vi "Lab Panel V4.91.vi"() -> ()   [LabVIEW 2013] (continued)
                            n2887 = case shown="True" w5366 {
                              tunnel: [w5368 0] -> w5364
                              tunnel: w5363 -> [w5368 _]
                              tunnel: w5365 -> [_ w5369]
                              frame False {
                              }
                              frame True {
                                n2888 = Concatenate Strings("LA02-1 ", w5369) -> (w5372:string)
                                n2889 = One Button Dialog(message=w5372) -> ()  [unwired: 1 in, 1 out]
                              }
                            }
                          }
                          frame #3 {
                            n2890 = Greater?(x=w5374, y=w5377) -> (0:w5376:bool)
                            n2891 = case shown="True" w5376 {
                              tunnel: [w5378 0] -> w5373
                              tunnel: w5374 -> [w5378 _]
                              tunnel: w5375 -> [_ w5379]
                              frame False {
                              }
                              frame True {
                                n2892 = Concatenate Strings("LA02-2 ", w5379) -> (w5382:string)
                                n2893 = One Button Dialog(message=w5382) -> ()  [unwired: 1 in, 1 out]
                              }
                            }
                          }
                          frame #4 {
                            n2894 = Greater?(x=w5384, y=w5387) -> (0:w5386:bool)
                            n2895 = case shown="True" w5386 {
                              tunnel: [w5388 0] -> w5383
                              tunnel: w5384 -> [w5388 _]
                              tunnel: w5385 -> [_ w5389]
                              frame False {
                              }
                              frame True {
                                n2896 = Concatenate Strings("LA03-1 ", w5389) -> (w5392:string)
                                n2897 = One Button Dialog(message=w5392) -> ()  [unwired: 1 in, 1 out]
                              }
                            }
                          }
                          frame #5 {
                            n2898 = Greater?(x=w5393, y=w5397) -> (0:w5396:bool)
                            n2899 = case shown="True" w5396 {
                              tunnel: [w5398 0] -> w5394
                              tunnel: w5393 -> [w5398 _]
                              tunnel: w5395 -> [_ w5399]
                              frame False {
                              }
                              frame True {
                                n2900 = Concatenate Strings("LA03-2 ", w5399) -> (w5402:string)
                                n2901 = One Button Dialog(message=w5402) -> ()  [unwired: 1 in, 1 out]
                              }
                            }
                          }
                          frame #6 {
                            n2902 = Greater?(x=w5404, y=w5407) -> (0:w5406:bool)
                            n2903 = case shown="True" w5406 {
                              tunnel: [w5408 0] -> w5403
                              tunnel: w5404 -> [w5408 _]
                              tunnel: w5405 -> [_ w5409]
                              frame False {
                              }
                              frame True {
                                n2904 = Concatenate Strings("LA04-1 ", w5409) -> (w5412:string)
                                n2905 = One Button Dialog(message=w5412) -> ()  [unwired: 1 in, 1 out]
                              }
                            }
                          }
                          frame #7 {
                            n2906 = Greater?(x=w5414, y=w5417) -> (0:w5416:bool)
                            n2907 = case shown="True" w5416 {
                              tunnel: [w5418 0] -> w5413
                              tunnel: w5414 -> [w5418 _]
                              tunnel: w5415 -> [_ w5419]
                              frame False {
                              }
                              frame True {
                                n2908 = Concatenate Strings("LA04-2 ", w5419) -> (w5422:string)
                                n2909 = One Button Dialog(message=w5422) -> ()  [unwired: 1 in, 1 out]
                              }
                            }
                          }
                          frame #8 {
                            n2910 = Greater?(x=w5424, y=w5427) -> (0:w5426:bool)
                            n2911 = case shown="True" w5426 {
                              tunnel: [w5428 0] -> w5423
                              tunnel: w5424 -> [w5428 _]
                              tunnel: w5425 -> [_ w5429]
                              frame False {
                              }
                              frame True {
                                n2912 = Concatenate Strings("LA05-1 ", w5429) -> (w5432:string)
                                n2913 = One Button Dialog(message=w5432) -> ()  [unwired: 1 in, 1 out]
                              }
                            }
                          }
                          frame #9 {
                            n2914 = Greater?(x=w5434, y=w5437) -> (0:w5436:bool)
                            n2915 = case shown="True" w5436 {
                              tunnel: [w5438 0] -> w5433
                              tunnel: w5434 -> [w5438 _]
                              tunnel: w5435 -> [_ w5439]
                              frame False {
                              }
                              frame True {
                                n2916 = Concatenate Strings("LA05-2 ", w5439) -> (w5442:string)
                                n2917 = One Button Dialog(message=w5442) -> ()  [unwired: 1 in, 1 out]
                              }
                            }
                          }
                        }
                        n2918 = Bundle By Name(cluster=w5341, "LAB01-1"=w5339, "LAB01-2"=w5337, "LAB02-1"=w5334, "LAB02-2"=w5331, "LAB03-1"=w5329, "LAB03-2"=w5328, "LAB04-1"=w5325, "LAB04-2"=w5323, "LAB05-1"=w5321, "LAB05-2"=w5319) -> (w5340:T8)
                        n2919 = local write "JIG RELAY CYCLES"(w5340) -> ()
                      }
                    }
                  }
                }
              }
            }
          }
          frame #19 {
            # "get temperature values"
            n2920 = local read "Panel #"() -> (w5443:dbl)
            n2921 = local read "simulate"() -> (w5456:bool)
            n2922 = local read "Temp Test Cal"() -> (w5453:dbl)
            n2923 = stacked-sequence {
              seq-local: [w5459 _] -> [_ w5495]
              tunnel: w5456 -> [_ w5509]
              tunnel: T14 {"1  (A) cal"=1.0, "1 (V) cal"=1.0, "1 (PF) cal"=1.0, "1 (TL) cal"=1.0, "1 (TN) cal"=1.0, "2 (A) cal"=1.0, "2 (V) cal"=1.0, "2 (PF) cal"=1.0, "2 (TL) cal"=1.0, "2 (TN) cal"=1.0} ("CAL LAB01") -> [_ w5508]
              tunnel: w5454 -> [_ w5507]
              tunnel: w5453 -> [_ w5506]
              tunnel: w5452 -> [_ w5505]
              tunnel: w5451 -> [_ w5504]
              tunnel: w5450 -> [_ w5503]
              tunnel: w5449 -> [_ w5502]
              tunnel: w5448 -> [_ w5501]
              tunnel: w5447 -> [_ w5500]
              tunnel: w5446 -> [_ w5499]
              tunnel: w5445 -> [_ w5498]
              tunnel: w5444 -> [_ w5497]
              tunnel: w5443 -> [_ w5496]
              frame #0 {
                n2924 = local read "Select COM port"() -> (w5460:refnum<visa-resource-name>)
                "COM port" <- w5460
                n2925 = global write "Global 1.vi" "COM port"(w5460) -> ()
                n2926 = global write "Global 1.vi" "tmp dly lps"("Temp Delay Lps") -> ()
                n2927 = global write "Global 1.vi" "dly value"("Temp Value") -> ()
                n2928 = local read "jig cycle"() -> (w5462:dbl)
                n2929 = local read "on loops"() -> (w5464:dbl)
                n2930 = Add(x=w5464, y=3) -> (x+y=w5465:dbl)
                n2931 = local read "Panel #"() -> (w5461:dbl)
                n2932 = Equal?(x=w5462, y=w5465) -> (x = y?=w5459:bool)
                n2933 = case shown="True" w5459 {
                  tunnel: w5461 -> [_ w5469]
                  frame False {
                  }
                  frame True {
                    n2934 = local read "simulate"() -> (w5466:bool)
                    n2935 = case shown="1" w5469 {
                      tunnel: 1.0 -> [_ w5474 w5476 w5482 w5486 w5491]
                      tunnel: w5466 -> [_ w5470 w5475 w5480 w5487 w5490]
                      frame 0, Default {
                      }
                      frame 1 {
                        w5472 = FALSE
                        n2936 = call "sub vi - GET ALL TEMP v6.vi"("LA01-EN"=TRUE, "simulate"=w5470, "LA02-EN"=w5472, "LA03-EN"=w5472, "LA04-EN"=w5472, "LA05-EN"=w5472, "Gen Cal Value"=w5474) -> ("LA01 TEMP"=w5471:T24)  [unwired: 3 in, 5 out]
                        n2937 = local write "LAB01 TEMP"(w5471) -> ()
                      }
                      frame 2 {
                        w5477 = FALSE
                        n2938 = call "sub vi - GET ALL TEMP v6.vi"("LA01-EN"=w5477, "simulate"=w5475, "LA02-EN"=TRUE, "LA03-EN"=w5477, "LA04-EN"=w5477, "LA05-EN"=w5477, "Gen Cal Value"=w5476) -> ("LA02 TEMP"=w5479:T24)  [unwired: 3 in, 5 out]
                        n2939 = local write "LAB02 TEMP"(w5479) -> ()
                      }
                      frame 3 {
                        w5483 = FALSE
                        n2940 = call "sub vi - GET ALL TEMP v6.vi"("LA01-EN"=w5483, "simulate"=w5480, "LA02-EN"=w5483, "LA03-EN"=TRUE, "LA04-EN"=w5483, "LA05-EN"=w5483, "Gen Cal Value"=w5482) -> ("LA03 TEMP"=w5481:T24)  [unwired: 3 in, 5 out]
                        n2941 = local write "LAB03 TEMP"(w5481) -> ()
                      }
                      frame 4 {
                        w5488 = FALSE
                        n2942 = call "sub vi - GET ALL TEMP v6.vi"("LA01-EN"=w5488, "simulate"=w5487, "LA02-EN"=w5488, "LA03-EN"=w5488, "LA04-EN"=TRUE, "LA05-EN"=w5488, "Gen Cal Value"=w5486) -> ("LA04 TEMP"=w5485:T24)  [unwired: 3 in, 5 out]
                        n2943 = local write "LAB04 TEMP"(w5485) -> ()
                      }
                      frame 5 {
                        w5493 = FALSE
                        n2944 = call "sub vi - GET ALL TEMP v6.vi"("LA01-EN"=w5493, "simulate"=w5490, "LA02-EN"=w5493, "LA03-EN"=w5493, "LA04-EN"=w5493, "LA05-EN"=TRUE, "Gen Cal Value"=w5491) -> ("LA05 TEMP"=w5492:T24)  [unwired: 3 in, 5 out]
                        n2945 = local write "LAB05 TEMP"(w5492) -> ()
                      }
                    }
                    n2946 = local write "TEMP"(TRUE) -> ()
                  }
                }
              }
              frame #1 {
                n2947 = case shown="True" w5495 {
                  tunnel: w5509 -> [_ w5523]
                  tunnel: w5508 -> [_ w5522]
                  tunnel: w5507 -> [_ w5521]
                  tunnel: w5506 -> [_ w5520]
                  tunnel: w5505 -> [_ w5519]
                  tunnel: w5504 -> [_ w5518]
                  tunnel: w5503 -> [_ w5517]
                  tunnel: w5502 -> [_ w5516]
                  tunnel: w5501 -> [_ w5515]
                  tunnel: w5500 -> [_ w5514]
                  tunnel: w5499 -> [_ w5513]
                  tunnel: w5498 -> [_ w5512]
                  tunnel: w5497 -> [_ w5511]
                  tunnel: w5496 -> [_ w5510]
                  frame False {
                  }
                  frame True {
                    n2948 = case shown="1" w5510 {
                      tunnel: w5523 -> [_ w5536 w5581 w5626 w5671 w5716]
                      tunnel: w5522 -> [_ w5535 w5580 w5625 w5670 w5715]
                      tunnel: w5521 -> [_ w5525 _ _ _ _]
                      tunnel: w5520 -> [_ w5530 w5579 w5624 w5669 w5714]
                      tunnel: w5519 -> [_ w5524 _ _ _ _]
                      tunnel: w5518 -> [_ _ w5570 _ _ _]
                      tunnel: w5517 -> [_ _ w5569 _ _ _]
                      tunnel: w5516 -> [_ _ _ w5615 _ _]
                      tunnel: w5515 -> [_ _ _ w5614 _ _]
                      tunnel: w5514 -> [_ _ _ _ w5660 _]
                      tunnel: w5513 -> [_ _ _ _ w5659 _]
                      tunnel: w5512 -> [_ _ _ _ _ w5705]
                      tunnel: w5511 -> [_ _ _ _ _ w5704]
                      frame ..0 {
                      }
                      frame 1 {
                        n2949 = case shown="False" w5536 {
                          tunnel: [w5567 w5568] -> w5552
                          tunnel: w5535 -> [_ w5568]
                          frame False {
                            n2950 = local read "CAL LAB01"() -> (w5567:T14)
                          }
                          frame True {
                          }
                        }
                        n2951 = local read "TEMP LA01"() -> (w5543:T9)
                        n2952 = local read "LAB01 TEMP"() -> (w5542:T12)
                        n2953 = call "sub vi - temperature delay v3.vi"("2-run"=w5524, "1-run"=w5525, "temp values IN"=w5543, "temp signals"=w5542) -> ("T2-N"=w5538:dbl, "T2-L"=w5539:dbl, "T1-N"=w5540:dbl, "T1-L"=w5541:dbl, "temp values OUT"=w5537:T43)  [unwired: 3 in]
                        n2954 = Unbundle By Name(w5552) -> ("1 (TL) cal"=w5547:dbl, "1 (TN) cal"=w5546:dbl, "2 (TL) cal"=w5545:dbl, "2 (TN) cal"=w5544:dbl)  [unwired: 6 out]
                        n2955 = local write "TEMP LA01"(w5537) -> ()
                        n2956 = Multiply(x=w5541, y=w5547) -> (x*y=w5534:dbl)
                        n2957 = Multiply(x=w5540, y=w5546) -> (x*y=w5532:dbl)
                        n2958 = Multiply(x=w5539, y=w5545) -> (x*y=w5529:dbl)
                        n2959 = Multiply(x=w5538, y=w5544) -> (x*y=w5528:dbl)
                        n2960 = case shown="True" w5525 {
                          tunnel: w5534 -> [w5561 w5566]
                          tunnel: w5530 -> [_ w5564]
                          tunnel: [w5561 w5565] -> w5533
                          tunnel: w5532 -> [w5560 w5563]
                          tunnel: [w5560 w5562] -> w5531
                          frame False {
                          }
                          frame True {
                            n2961 = Multiply(x=w5564, y=w5563) -> (x*y=w5562:dbl)
                            n2962 = Multiply(x=w5564, y=w5566) -> (x*y=w5565:dbl)
                          }
                        }
                        n2963 = case shown="True" w5524 {
                          tunnel: w5529 -> [w5554 w5559]
                          tunnel: w5530 -> [_ w5557]
                          tunnel: [w5554 w5558] -> w5527
                          tunnel: w5528 -> [w5553 w5556]
                          tunnel: [w5553 w5555] -> w5526
                          frame False {
                          }
                          frame True {
                            n2964 = Multiply(x=w5557, y=w5556) -> (x*y=w5555:dbl)
                            n2965 = Multiply(x=w5557, y=w5559) -> (x*y=w5558:dbl)
                          }
                        }
                        n2966 = local read "SIG LAB01-2"() -> (w5549:T2)
                        n2967 = local read "SIG LAB01-1"() -> (w5551:T2)
                        n2968 = Bundle By Name(cluster=w5551, "Tmp Live"=w5533, "Tmp Neut"=w5531) -> (w5550:T2)
                        n2969 = Bundle By Name(cluster=w5549, "Tmp Live"=w5527, "Tmp Neut"=w5526) -> (w5548:T2)
                        n2970 = local write "SIG LAB01-1"(w5550) -> ()
                        n2971 = local write "SIG LAB01-2"(w5548) -> ()
                      }
                      frame 2 {
                        n2972 = case shown="True" w5581 {
                          tunnel: [w5612 w5613] -> w5597
                          tunnel: w5580 -> [_ w5613]
                          frame False {
                            n2973 = local read "CAL LAB02"() -> (w5612:T15)
                          }
                          frame True {
                          }
                        }
                        n2974 = local read "LAB02 TEMP"() -> (w5588:T12)
                        n2975 = local read "TEMP LA02"() -> (w5587:T9)
                        n2976 = call "sub vi - temperature delay v3.vi"("2-run"=w5569, "1-run"=w5570, "temp values IN"=w5587, "temp signals"=w5588) -> ("T2-N"=w5582:dbl, "T2-L"=w5583:dbl, "T1-N"=w5584:dbl, "T1-L"=w5585:dbl, "temp values OUT"=w5586:T43)  [unwired: 3 in]
                        n2977 = Unbundle By Name(w5597) -> ("1 (TL) cal"=w5592:dbl, "1 (TN) cal"=w5591:dbl, "2 (TL) cal"=w5590:dbl, "2 (TN) cal"=w5589:dbl)  [unwired: 6 out]
                        n2978 = local write "TEMP LA02"(w5586) -> ()
                        n2979 = Multiply(x=w5585, y=w5592) -> (x*y=w5578:dbl)
                        n2980 = Multiply(x=w5584, y=w5591) -> (x*y=w5577:dbl)
                        n2981 = Multiply(x=w5583, y=w5590) -> (x*y=w5574:dbl)
                        n2982 = Multiply(x=w5582, y=w5589) -> (x*y=w5573:dbl)
                        n2983 = case shown="True" w5570 {
                          tunnel: w5578 -> [w5606 w5611]
                          tunnel: w5579 -> [_ w5609]
                          tunnel: [w5606 w5610] -> w5576
                          tunnel: w5577 -> [w5605 w5608]
                          tunnel: [w5605 w5607] -> w5575
                          frame False {
                          }
                          frame True {
                            n2984 = Multiply(x=w5609, y=w5608) -> (x*y=w5607:dbl)
                            n2985 = Multiply(x=w5609, y=w5611) -> (x*y=w5610:dbl)
                          }
                        }
                        n2986 = case shown="True" w5569 {
                          tunnel: w5574 -> [w5599 w5604]
                          tunnel: w5579 -> [_ w5602]
                          tunnel: [w5599 w5603] -> w5572
                          tunnel: w5573 -> [w5598 w5601]
                          tunnel: [w5598 w5600] -> w5571
                          frame False {
                          }
                          frame True {
                            n2987 = Multiply(x=w5602, y=w5601) -> (x*y=w5600:dbl)
                            n2988 = Multiply(x=w5602, y=w5604) -> (x*y=w5603:dbl)
                          }
                        }
                        n2989 = local read "SIG LAB02-2"() -> (w5594:T2)
                        n2990 = local read "SIG LAB02-1"() -> (w5596:T2)
                        n2991 = Bundle By Name(cluster=w5596, "Tmp Live"=w5576, "Tmp Neut"=w5575) -> (w5595:T2)
                        n2992 = Bundle By Name(cluster=w5594, "Tmp Live"=w5572, "Tmp Neut"=w5571) -> (w5593:T2)
                        n2993 = local write "SIG LAB02-1"(w5595) -> ()
                        n2994 = local write "SIG LAB02-2"(w5593) -> ()
                      }
                      frame 3 {
                        n2995 = case shown="False" w5626 {
                          tunnel: [w5657 w5658] -> w5642
                          tunnel: w5625 -> [_ w5658]
                          frame False {
                            n2996 = local read "CAL LAB03"() -> (w5657:T14)
                          }
                          frame True {
                          }
                        }
                        n2997 = local read "TEMP LA03"() -> (w5632:T9)
                        n2998 = local read "LAB03 TEMP"() -> (w5633:T12)
                        n2999 = call "sub vi - temperature delay v3.vi"("2-run"=w5614, "1-run"=w5615, "temp values IN"=w5632, "temp signals"=w5633) -> ("T2-N"=w5627:dbl, "T2-L"=w5628:dbl, "T1-N"=w5629:dbl, "T1-L"=w5630:dbl, "temp values OUT"=w5631:T43)  [unwired: 3 in]
                        n3000 = Unbundle By Name(w5642) -> ("1 (TL) cal"=w5637:dbl, "1 (TN) cal"=w5636:dbl, "2 (TL) cal"=w5635:dbl, "2 (TN) cal"=w5634:dbl)  [unwired: 6 out]
                        n3001 = local write "TEMP LA03"(w5631) -> ()
                        n3002 = Multiply(x=w5630, y=w5637) -> (x*y=w5623:dbl)
                        n3003 = Multiply(x=w5629, y=w5636) -> (x*y=w5622:dbl)
                        n3004 = Multiply(x=w5628, y=w5635) -> (x*y=w5619:dbl)
                        n3005 = Multiply(x=w5627, y=w5634) -> (x*y=w5618:dbl)
                        n3006 = case shown="True" w5614 {
                          tunnel: w5619 -> [w5644 w5649]
                          tunnel: w5624 -> [_ w5647]
                          tunnel: [w5644 w5648] -> w5617
                          tunnel: w5618 -> [w5643 w5646]
                          tunnel: [w5643 w5645] -> w5616
                          frame False {
                          }
                          frame True {
                            n3007 = Multiply(x=w5647, y=w5646) -> (x*y=w5645:dbl)
                            n3008 = Multiply(x=w5647, y=w5649) -> (x*y=w5648:dbl)
                          }
                        }
                        n3009 = case shown="True" w5615 {
                          tunnel: w5623 -> [w5651 w5656]
                          tunnel: w5624 -> [_ w5654]
                          tunnel: [w5651 w5655] -> w5621
                          tunnel: w5622 -> [w5650 w5653]
                          tunnel: [w5650 w5652] -> w5620
                          frame False {
                          }
                          frame True {
                            n3010 = Multiply(x=w5654, y=w5653) -> (x*y=w5652:dbl)
                            n3011 = Multiply(x=w5654, y=w5656) -> (x*y=w5655:dbl)
                          }
                        }
                        n3012 = local read "SIG LAB03-2"() -> (w5639:T2)
                        n3013 = local read "SIG LAB03-1"() -> (w5641:T2)
                        n3014 = Bundle By Name(cluster=w5641, "Tmp Live"=w5621, "Tmp Neut"=w5620) -> (w5640:T2)
                        n3015 = Bundle By Name(cluster=w5639, "Tmp Live"=w5617, "Tmp Neut"=w5616) -> (w5638:T2)
                        n3016 = local write "SIG LAB03-1"(w5640) -> ()
                        n3017 = local write "SIG LAB03-2"(w5638) -> ()
                      }
                      frame 4 {
                        n3018 = case shown="False" w5671 {
                          tunnel: [w5702 w5703] -> w5687
                          tunnel: w5670 -> [_ w5703]
                          frame False {
                            n3019 = local read "CAL LAB04"() -> (w5702:T14)
                          }
                          frame True {
                          }
                        }
                        n3020 = local read "LAB04 TEMP"() -> (w5677:T12)
                        n3021 = local read "TEMP LA04"() -> (w5678:T9)
                        n3022 = call "sub vi - temperature delay v3.vi"("2-run"=w5659, "1-run"=w5660, "temp values IN"=w5678, "temp signals"=w5677) -> ("T2-N"=w5672:dbl, "T2-L"=w5673:dbl, "T1-N"=w5674:dbl, "T1-L"=w5675:dbl, "temp values OUT"=w5676:T43)  [unwired: 3 in]
                        n3023 = Unbundle By Name(w5687) -> ("1 (TL) cal"=w5682:dbl, "1 (TN) cal"=w5681:dbl, "2 (TL) cal"=w5680:dbl, "2 (TN) cal"=w5679:dbl)  [unwired: 6 out]
                        n3024 = local write "TEMP LA04"(w5676) -> ()
                        n3025 = Multiply(x=w5675, y=w5682) -> (x*y=w5668:dbl)
                        n3026 = Multiply(x=w5674, y=w5681) -> (x*y=w5667:dbl)
                        n3027 = Multiply(x=w5673, y=w5680) -> (x*y=w5664:dbl)
                        n3028 = Multiply(x=w5672, y=w5679) -> (x*y=w5663:dbl)
                        n3029 = case shown="True" w5659 {
                          tunnel: w5664 -> [w5689 w5694]
                          tunnel: w5669 -> [_ w5692]
                          tunnel: [w5689 w5693] -> w5662
                          tunnel: w5663 -> [w5688 w5691]
                          tunnel: [w5688 w5690] -> w5661
                          frame False {
                          }
                          frame True {
                            n3030 = Multiply(x=w5692, y=w5691) -> (x*y=w5690:dbl)
                            n3031 = Multiply(x=w5692, y=w5694) -> (x*y=w5693:dbl)
                          }
                        }
                        n3032 = case shown="True" w5660 {
                          tunnel: w5668 -> [w5696 w5701]
                          tunnel: w5669 -> [_ w5699]
                          tunnel: [w5696 w5700] -> w5666
                          tunnel: w5667 -> [w5695 w5698]
                          tunnel: [w5695 w5697] -> w5665
                          frame False {
                          }
                          frame True {
                            n3033 = Multiply(x=w5699, y=w5698) -> (x*y=w5697:dbl)
                            n3034 = Multiply(x=w5699, y=w5701) -> (x*y=w5700:dbl)
                          }
                        }
                        n3035 = local read "SIG LAB04-2"() -> (w5684:T2)
                        n3036 = local read "SIG LAB04-1"() -> (w5686:T2)
                        n3037 = Bundle By Name(cluster=w5686, "Tmp Live"=w5666, "Tmp Neut"=w5665) -> (w5685:T2)
                        n3038 = Bundle By Name(cluster=w5684, "Tmp Live"=w5662, "Tmp Neut"=w5661) -> (w5683:T2)
                        n3039 = local write "SIG LAB04-1"(w5685) -> ()
                        n3040 = local write "SIG LAB04-2"(w5683) -> ()
                      }
                      frame 5.. {
                        n3041 = case shown="False" w5716 {
                          tunnel: [w5747 w5748] -> w5732
                          tunnel: w5715 -> [_ w5748]
                          frame False {
                            n3042 = local read "CAL LAB05"() -> (w5747:T14)
                          }
                          frame True {
                          }
                        }
                        n3043 = local read "LAB05 TEMP"() -> (w5722:T12)
                        n3044 = local read "TEMP LA05"() -> (w5723:T9)
                        n3045 = call "sub vi - temperature delay v3.vi"("2-run"=w5704, "1-run"=w5705, "temp values IN"=w5723, "temp signals"=w5722) -> ("T2-N"=w5718:dbl, "T2-L"=w5719:dbl, "T1-N"=w5720:dbl, "T1-L"=w5721:dbl, "temp values OUT"=w5717:T43)  [unwired: 3 in]
                        n3046 = local write "TEMP LA05"(w5717) -> ()
                        n3047 = Unbundle By Name(w5732) -> ("1 (TL) cal"=w5724:dbl, "1 (TN) cal"=w5727:dbl, "2 (TL) cal"=w5726:dbl, "2 (TN) cal"=w5725:dbl)  [unwired: 6 out]
                        n3048 = Multiply(x=w5721, y=w5724) -> (x*y=w5713:dbl)
                        n3049 = Multiply(x=w5720, y=w5727) -> (x*y=w5712:dbl)
                        n3050 = Multiply(x=w5719, y=w5726) -> (x*y=w5709:dbl)
                        n3051 = Multiply(x=w5718, y=w5725) -> (x*y=w5708:dbl)
                        n3052 = case shown="True" w5704 {
                          tunnel: w5709 -> [w5734 w5739]
                          tunnel: w5714 -> [_ w5737]
                          tunnel: [w5734 w5738] -> w5707
                          tunnel: w5708 -> [w5733 w5736]
                          tunnel: [w5733 w5735] -> w5706
                          frame False {
                          }
                          frame True {
                            n3053 = Multiply(x=w5737, y=w5736) -> (x*y=w5735:dbl)
                            n3054 = Multiply(x=w5737, y=w5739) -> (x*y=w5738:dbl)
                          }
                        }
                        n3055 = case shown="True" w5705 {
                          tunnel: w5713 -> [w5741 w5746]
                          tunnel: w5714 -> [_ w5744]
                          tunnel: [w5741 w5745] -> w5711
                          tunnel: w5712 -> [w5740 w5743]
                          tunnel: [w5740 w5742] -> w5710
                          frame False {
                          }
                          frame True {
                            n3056 = Multiply(x=w5744, y=w5743) -> (x*y=w5742:dbl)
                            n3057 = Multiply(x=w5744, y=w5746) -> (x*y=w5745:dbl)
                          }
                        }
                        n3058 = local read "SIG LAB05-1"() -> (w5731:T2)
                        n3059 = Bundle By Name(cluster=w5731, "Tmp Live"=w5711, "Tmp Neut"=w5710) -> (w5730:T2)
                        n3060 = local read "SIG LAB05-2"() -> (w5729:T2)
                        n3061 = Bundle By Name(cluster=w5729, "Tmp Live"=w5707, "Tmp Neut"=w5706) -> (w5728:T2)
                        n3062 = local write "SIG LAB05-1"(w5730) -> ()
                        n3063 = local write "SIG LAB05-2"(w5728) -> ()
                      }
                    }
                  }
                }
              }
            }
          }
          frame #20 {
            # "write data to display panel"
            n3064 = global write "Global display 1.vi" "TEST 5-2"(w5783) -> ()
            n3065 = global write "Global display 1.vi" "TEST 4-2"(w5785) -> ()
            n3066 = global write "Global display 1.vi" "TEST 1-2"(w5791) -> ()
            n3067 = global write "Global display 1.vi" "TEST 3-1"(w5788) -> ()
            n3068 = global write "Global display 1.vi" "TEST 5-1"(w5784) -> ()
            n3069 = global write "Global display 1.vi" "TEST 1-1"(w5792) -> ()
            n3070 = global write "Global display 1.vi" "TEST 3-2"(w5787) -> ()
            n3071 = global write "Global display 1.vi" "TEST 4-1"(w5786) -> ()
            n3072 = global write "Global display 1.vi" "TEST 2-2"(w5789) -> ()
            n3073 = global write "Global display 1.vi" "TEST 2-1"(w5790) -> ()
            n3074 = global read "Global display 3.vi" "log 1-1"() -> (→"LOG LAB01-1":string)
            n3075 = global read "Global display 3.vi" "log 3-1"() -> (→"LOG LAB03-1":string)
            n3076 = global read "Global display 3.vi" "log 1-2"() -> (→"LOG LAB01-2":string)
            n3077 = property on="Tab Control 2" class="TabCtl (strict)"() -> ("Pages"=w5782:refnum<vi>[])  [unwired: 2 in, 2 out]
            n3078 = global read "Global display 3.vi" "log 2-1"() -> (→"LOG LAB02-1":string)
            n3079 = global read "Global display 3.vi" "log 2-2"() -> (→"LOG LAB02-2":string)
            n3080 = global read "Global display 3.vi" "log 4-2"() -> (→"LOG LAB04-2":string)
            n3081 = global read "Global display 3.vi" "log 5-2"() -> (→"LOG LAB05-2":string)
            n3082 = global read "Global display 3.vi" "log 5-1"() -> (→"LOG LAB05-1":string)
            n3083 = global read "Global display 3.vi" "log 4-1"() -> (→"LOG LAB04-1":string)
            n3084 = global read "Global display 3.vi" "log 3-2"() -> (→"LOG LAB03-2":string)
            n3085 = Index Array(array=w5782, index=8) -> (element=w5780:refnum<vi>)
            n3086 = property class="Page"(reference=w5780) -> ("PageVis"=w5779:bool)  [unwired: 1 in, 2 out]
            n3087 = global write "Global display 3.vi" "admin"(w5779) -> ()
            n3088 = local read "O/I  LAB05-2"() -> (w5833:bool)
            n3089 = local read "O/I  LAB05-1"() -> (w5834:bool)
            n3090 = local read "O/I  LAB03-2"() -> (w5837:bool)
            n3091 = local read "O/I  LAB04-2"() -> (w5835:bool)
            n3092 = local read "O/I  LAB04-1"() -> (w5836:bool)
            n3093 = local read "O/I  LAB03-1"() -> (w5838:bool)
            n3094 = local read "O/I  LAB01-2"() -> (w5841:bool)
            n3095 = local read "O/I  LAB01-1"() -> (w5842:bool)
            n3096 = local read "O/I  LAB02-1"() -> (w5840:bool)
            n3097 = local read "O/I  LAB02-2"() -> (w5839:bool)
            n3098 = global write "Global display 1.vi" "5-2 O/F"(w5833) -> ()
            n3099 = global write "Global display 1.vi" "5-1 O/F"(w5834) -> ()
            n3100 = global write "Global display 1.vi" "4-1 O/F"(w5836) -> ()
            n3101 = global write "Global display 1.vi" "4-2 O/F"(w5835) -> ()
            n3102 = global write "Global display 1.vi" "3-2 O/F"(w5837) -> ()
            n3103 = global write "Global display 1.vi" "3-1 O/F"(w5838) -> ()
            n3104 = global write "Global display 1.vi" "2-2 O/F"(w5839) -> ()
            n3105 = global write "Global display 1.vi" "2-1 O/F"(w5840) -> ()
            n3106 = global write "Global display 1.vi" "1-2 O/F"(w5841) -> ()
            n3107 = global write "Global display 1.vi" "1-1 O/F"(w5842) -> ()
            n3108 = local read "TEMP START LAB02-2"() -> (w5765:cluster{"TL":dbl, "TN":dbl})
            n3109 = local read "run lab05-2"() -> (w5823:bool)
            n3110 = local read "TEMP START LAB01-2"() -> (w5767:cluster{"TL":dbl, "TN":dbl})
            n3111 = local read "TEMP START LAB02-1"() -> (w5766:cluster{"TL":dbl, "TN":dbl})
            n3112 = local read "TEMP START LAB04-1"() -> (w5762:cluster{"TL":dbl, "TN":dbl})
            n3113 = local read "TEMP START LAB04-2"() -> (w5761:cluster{"TL":dbl, "TN":dbl})
            n3114 = local read "run lab04-1"() -> (w5826:bool)
            n3115 = local read "run lab04-2"() -> (w5825:bool)
            n3116 = local read "run lab05-1"() -> (w5824:bool)
            n3117 = local read "TEMP START LAB01-1"() -> (w5768:cluster{"TL":dbl, "TN":dbl})
            n3118 = local read "TEMP START LAB05-2"() -> (w5759:cluster{"TL":dbl, "TN":dbl})
            n3119 = local read "TEMP START LAB05-1"() -> (w5760:cluster{"TL":dbl, "TN":dbl})
            n3120 = local read "run lab03-2"() -> (w5827:bool)
            n3121 = local read "TEMP START LAB03-2"() -> (w5763:cluster{"TL":dbl, "TN":dbl})
            n3122 = local read "TEMP START LAB03-1"() -> (w5764:cluster{"TL":dbl, "TN":dbl})
            n3123 = local read "run lab02-1"() -> (w5830:bool)
            n3124 = local read "run lab03-1"() -> (w5828:bool)
            n3125 = local read "run lab01-2"() -> (w5831:bool)
            n3126 = local read "run lab02-2"() -> (w5829:bool)
            n3127 = local read "run lab01-1"() -> (w5832:bool)
            n3128 = global write "Global display 1.vi" "5-2 R/S"(w5823) -> ()
            n3129 = global write "Global display 1.vi" "5-1 R/S"(w5824) -> ()
            n3130 = global write "Global display 1.vi" "4-2 R/S"(w5825) -> ()
            n3131 = global write "Global display 1.vi" "4-1 R/S"(w5826) -> ()
            n3132 = global write "Global display 1.vi" "3-2 R/S"(w5827) -> ()
            n3133 = global write "Global display 1.vi" "1-2 R/S"(w5831) -> ()
            n3134 = global write "Global display 1.vi" "2-1 R/S"(w5830) -> ()
            n3135 = global write "Global display 1.vi" "3-1 R/S"(w5828) -> ()
            n3136 = global write "Global display 1.vi" "2-2 R/S"(w5829) -> ()
            n3137 = global write "Global display 1.vi" "1-1 R/S"(w5832) -> ()
            n3138 = global write "Global display 3.vi" "TEMP ST 05-2"(w5759) -> ()
            n3139 = global write "Global display 3.vi" "TEMP ST 05-1"(w5760) -> ()
            n3140 = global write "Global display 3.vi" "TEMP ST 03-2"(w5763) -> ()
            n3141 = global write "Global display 3.vi" "TEMP ST 04-2"(w5761) -> ()
            n3142 = global write "Global display 3.vi" "TEMP ST 01-1"(w5768) -> ()
            n3143 = global write "Global display 3.vi" "TEMP ST 01-2"(w5767) -> ()
            n3144 = global write "Global display 3.vi" "TEMP ST 04-1"(w5762) -> ()
            n3145 = global write "Global display 3.vi" "TEMP ST 02-1"(w5766) -> ()
            n3146 = global write "Global display 3.vi" "TEMP ST 02-2"(w5765) -> ()
            n3147 = global write "Global display 3.vi" "TEMP ST 03-1"(w5764) -> ()
            n3148 = local read "DISP LAB04-2"() -> (w5815:T4)
            n3149 = local read "DISP LAB05-1"() -> (w5814:T4)
            n3150 = local read "DISP LAB04-1"() -> (w5816:T4)
            n3151 = local read "DISP LAB05-2"() -> (w5813:T4)
            n3152 = local read "DISP LAB03-1"() -> (w5818:T4)
            n3153 = local read "DISP LAB03-2"() -> (w5817:T4)
            n3154 = local read "DISP LAB01-2"() -> (w5821:T4)
            n3155 = local read "DISP LAB02-1"() -> (w5820:T4)
            n3156 = local read "DISP LAB02-2"() -> (w5819:T4)
            n3157 = local read "DISP LAB01-1"() -> (w5822:T4)
            n3158 = local read "TEMP RISE LAB05-1"() -> (w5750:cluster{"TL":dbl, "TN":dbl})
            n3159 = local read "TEMP RISE LAB05-2"() -> (w5749:cluster{"TL":dbl, "TN":dbl})
            n3160 = local read "TEMP RISE LAB04-2"() -> (w5751:cluster{"TL":dbl, "TN":dbl})
            n3161 = local read "TEMP RISE LAB04-1"() -> (w5752:cluster{"TL":dbl, "TN":dbl})
            n3162 = local read "TEMP RISE LAB03-2"() -> (w5753:cluster{"TL":dbl, "TN":dbl})
            n3163 = local read "TEMP RISE LAB03-1"() -> (w5754:cluster{"TL":dbl, "TN":dbl})
            n3164 = local read "TEMP RISE LAB01-2"() -> (w5757:cluster{"TL":dbl, "TN":dbl})
            n3165 = local read "TEMP RISE LAB02-2"() -> (w5755:cluster{"TL":dbl, "TN":dbl})
            n3166 = local read "TEMP RISE LAB01-1"() -> (w5758:cluster{"TL":dbl, "TN":dbl})
            n3167 = local read "TEMP RISE LAB02-1"() -> (w5756:cluster{"TL":dbl, "TN":dbl})
            n3168 = global write "Global display 2.vi" "DISP LAB05-1"(w5814) -> ()
            n3169 = global write "Global display 2.vi" "DISP LAB05-2"(w5813) -> ()
            n3170 = global write "Global display 2.vi" "DISP LAB04-2"(w5815) -> ()
            n3171 = global write "Global display 2.vi" "DISP LAB02-1"(w5820) -> ()
            n3172 = global write "Global display 2.vi" "DISP LAB02-2"(w5819) -> ()
            n3173 = global write "Global display 2.vi" "DISP LAB04-1"(w5816) -> ()
            n3174 = global write "Global display 2.vi" "DISP LAB01-2"(w5821) -> ()
            n3175 = global write "Global display 2.vi" "DISP LAB01-1"(w5822) -> ()
            n3176 = global write "Global display 2.vi" "DISP LAB03-1"(w5818) -> ()
            n3177 = global write "Global display 2.vi" "DISP LAB03-2"(w5817) -> ()
            n3178 = global write "Global display 3.vi" "TEMP RS 05-2"(w5749) -> ()
            n3179 = global write "Global display 3.vi" "TEMP RS 05-1"(w5750) -> ()
            n3180 = global write "Global display 3.vi" "TEMP RS 03-2"(w5753) -> ()
            n3181 = global write "Global display 3.vi" "TEMP RS 02-1"(w5756) -> ()
            n3182 = global write "Global display 3.vi" "TEMP RS 02-2"(w5755) -> ()
            n3183 = global write "Global display 3.vi" "TEMP RS 04-2"(w5751) -> ()
            n3184 = global write "Global display 3.vi" "TEMP RS 01-2"(w5757) -> ()
            n3185 = global write "Global display 3.vi" "TEMP RS 03-1"(w5754) -> ()
            n3186 = global write "Global display 3.vi" "TEMP RS 04-1"(w5752) -> ()
            n3187 = global write "Global display 3.vi" "TEMP RS 01-1"(w5758) -> ()
            n3188 = local read "SET LAB05-2"() -> (w5803:T5)
            n3189 = local read "SET LAB05-1"() -> (w5804:T5)
            n3190 = local read "SET LAB04-1"() -> (w5806:T5)
            n3191 = local read "SET LAB04-2"() -> (w5805:T5)
            n3192 = local read "SET LAB03-1"() -> (w5808:T5)
            n3193 = local read "SET LAB03-2"() -> (w5807:T5)
            n3194 = local read "SET LAB02-2"() -> (w5809:T5)
            n3195 = local read "SET LAB01-2"() -> (w5811:T5)
            n3196 = local read "SET LAB02-1"() -> (w5810:T5)
            n3197 = local read "SET LAB01-1"() -> (w5812:T5)
            n3198 = global write "Global display 2.vi" "SET LAB05-2"(w5803) -> ()
            n3199 = global write "Global display 2.vi" "SET LAB05-1"(w5804) -> ()
            n3200 = global write "Global display 2.vi" "SET LAB04-1"(w5806) -> ()
            n3201 = global write "Global display 2.vi" "SET LAB04-2"(w5805) -> ()
            n3202 = global write "Global display 2.vi" "SET LAB03-2"(w5807) -> ()
            n3203 = global write "Global display 2.vi" "SET LAB02-2"(w5809) -> ()
            n3204 = global write "Global display 2.vi" "SET LAB03-1"(w5808) -> ()
            n3205 = global write "Global display 2.vi" "SET LAB01-2"(w5811) -> ()
            n3206 = global write "Global display 2.vi" "SET LAB01-1"(w5812) -> ()
            n3207 = global write "Global display 2.vi" "SET LAB02-1"(w5810) -> ()
            n3208 = local read "RESULT LAB01-1"() -> (w5802:bool)
            n3209 = local read "RESULT LAB03-2"() -> (w5797:bool)
            n3210 = local read "RESULT LAB04-1"() -> (w5796:bool)
            n3211 = local read "RESULT LAB04-2"() -> (w5795:bool)
            n3212 = local read "RESULT LAB02-2"() -> (w5799:bool)
            n3213 = local read "RESULT LAB01-2"() -> (w5801:bool)
            n3214 = local read "RESULT LAB02-1"() -> (w5800:bool)
            n3215 = local read "RESULT LAB03-1"() -> (w5798:bool)
            n3216 = local read "RESULT LAB05-1"() -> (w5794:bool)
            n3217 = local read "RESULT LAB05-2"() -> (w5793:bool)
            n3218 = global write "Global display 2.vi" "RESULT LAB05-1"(w5794) -> ()
            n3219 = global write "Global display 2.vi" "RESULT LAB01-2"(w5801) -> ()
            n3220 = global write "Global display 2.vi" "RESULT LAB03-2"(w5797) -> ()
            n3221 = global write "Global display 2.vi" "RESULT LAB04-1"(w5796) -> ()
            n3222 = global write "Global display 2.vi" "RESULT LAB04-2"(w5795) -> ()
            n3223 = global write "Global display 2.vi" "RESULT LAB05-2"(w5793) -> ()
            n3224 = global write "Global display 2.vi" "RESULT LAB03-1"(w5798) -> ()
            n3225 = global write "Global display 2.vi" "RESULT LAB02-1"(w5800) -> ()
            n3226 = global write "Global display 2.vi" "RESULT LAB02-2"(w5799) -> ()
            n3227 = global write "Global display 2.vi" "RESULT LAB01-1"(w5802) -> ()
          }
          frame #21 {
            # "simulate values"
            n3228 = global write "Global display 4.vi" "LAB deg C"("LAB deg C") -> ()
          }
          frame #22 {
            # "end main and display program"
            n3229 = Quit LabVIEW(quit? (T)="stop all") -> ()
            n3230 = global write "Global display 1.vi" "stop disp"("stop all") -> ()
          }
        }
        n3231 = node-c288() -> ()  [unwired: 1 in, 1 out]
        "loops" <- w312
      }
      n3232 = node-c288(w289) -> ()  [unwired: 1 out]
    }
  }
